vi "Dispose Report.vi"(0 "report in":refnum<class "NI_HTML.lvclass">, 5 "wait until printing completed? (T)":bool=TRUE, 9 "save changes? (F)":bool, 11 "error in (no error)":errorcluster, 12 "close report? (T)":bool=TRUE) -> (15 "error out":errorcluster)   [LabVIEW 2020, in "NI_HTML.lvclass"]
doc: "Closes the report and releases its interface, which saves memory."
uses:
  NI_HTML.lvclass
  NI_HTML.lvclass/NI_HTML.ctl
  NI_ReportGenerationCore.lvlib
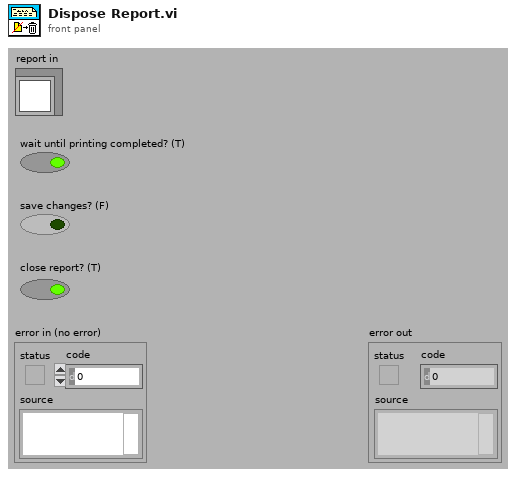
[diagram p1: front panel]
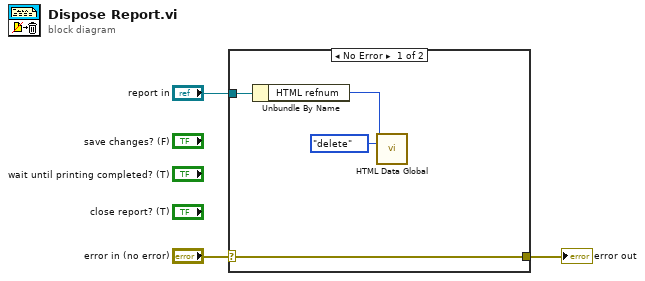
[diagram p0: block diagram]
diagram:
  n1 = case shown="No Error" "error in (no error)" {
    selector: "error in (no error)" -> [w7 w8]
    tunnel: [w7 w8] -> w2
    tunnel: "report in" -> [w6 _]
    frame No Error {
      n2 = Unbundle By Name(w6) -> ("HTML refnum"=w5:u32)
      n3 = call "HTML Data Global.vi"("HTML refnum"=w5, "menu"=enum16{"init", "get", "set", "delete"}."delete") -> ()  [unwired: 1 in, 13 out]
    }
    frame Error {
    }
  }
  "error out" <- w2
